vi "Set acceleration DSP402.vi"(8 "error in (no error)":errorcluster, 10 "Acceleration units":u32, 11 "DSP402 in":refnum<class "DSP402.lvclass">) -> (0 "error out":errorcluster, 3 "DSP402 out":refnum<class "DSP402.lvclass">)   [LabVIEW 2017, in "canopen.lvlib" / "DSP402.lvclass"]
uses:
  DSP402.lvclass
  DSP402.lvclass/DSP402.ctl
  CANopen/Multiplexor.ctl
  Download DSP402 (U32).vi
  CANopen/CANopen.lvclass
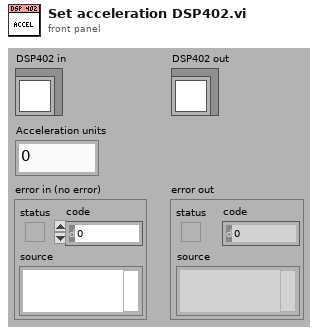
[diagram p1: front panel]
types:
  T1 = typedef "canopen.lvlib/DSP402.lvclass/DriveMode.ctl" = i8
  T2 = typedef "canopen.lvlib/CANopen.lvclass/Multiplexor.ctl" = cluster{"Index":u16, "Sub-index":u8}
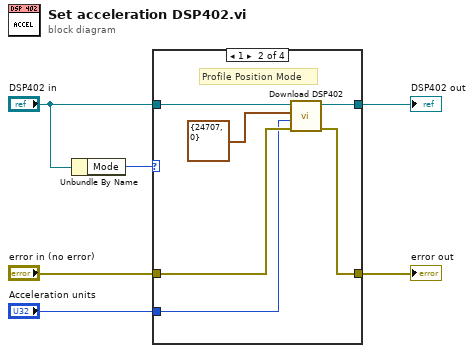
[diagram p0: block diagram]
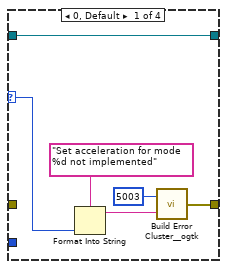
[diagram p2: hidden frame]
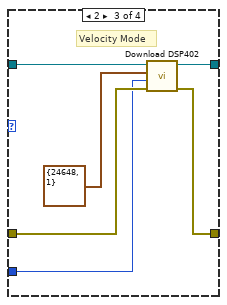
[diagram p3: hidden frame]
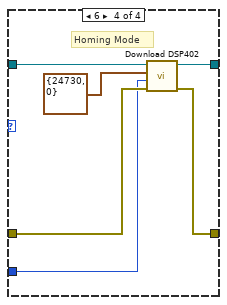
[diagram p4: hidden frame]
diagram:
  n1 = Unbundle By Name("DSP402 in") -> ("Mode"=w3:T1)
  n2 = case shown="1" w3 {
    selector: w3 -> [w9 _ _ _]
    tunnel: [w10 w17 w23 w29] -> w4
    tunnel: "error in (no error)" -> [_ w16 w22 w28]
    tunnel: "Acceleration units" -> [_ w15 w21 w27]
    tunnel: [w7 w13 w19 w25] -> w2
    tunnel: "DSP402 in" -> [w7 w14 w20 w26]
    frame 0, Default {
      n3 = Format Into String(format string="Set acceleration for mode %d not implemented", w9) -> (resulting string=w11:string)  [unwired: 2 in, 1 out]
      n4 = call <userlib>:"Build Error Cluster__ogtk.vi"("String to Prepend to source (\"\")"=w11, "code"=5003) -> ("error out"=w10:errorcluster)
    }
    frame 1 {
      # "Profile Position Mode"
      n5 = call-poly "Download DSP402.vi"("error in (no error)"=w16, "Value"=w15, "Multiplexor"=T2 {"Index"=24707, "Sub-index"=0}, "DSP402 in"=w14) -> ("error out"=w17:errorcluster, "DSP402 out"=w13:refnum<class "DSP402.lvclass">)  [unwired: 1 in, 1 out]
    }
    frame 2 {
      # "Velocity Mode"
      n6 = call-poly "Download DSP402.vi"("error in (no error)"=w22, "Value"=w21, "Multiplexor"=T2 {"Index"=24648, "Sub-index"=1}, "DSP402 in"=w20) -> ("error out"=w23:errorcluster, "DSP402 out"=w19:refnum<class "DSP402.lvclass">)  [unwired: 2 out]
    }
    frame 6 {
      # "Homing Mode"
      n7 = call-poly "Download DSP402.vi"("error in (no error)"=w28, "Value"=w27, "Multiplexor"=T2 {"Index"=24730, "Sub-index"=0}, "DSP402 in"=w26) -> ("error out"=w29:errorcluster, "DSP402 out"=w25:refnum<class "DSP402.lvclass">)  [unwired: 1 in, 1 out]
    }
  }
  "error out" <- w4
  "DSP402 out" <- w2
